vi "Main Generador N01.vi"(8 "error in":errorcluster, 11 "Network Path":string="192.168.169.1") -> (0 "error out":errorcluster, 2 "Equipo conectado":bool)   [LabVIEW 2018]
panel:
  out "current time":timestamp
  in  "Stop Button":bool
  out "Alarmas":string
  out "I3_IEE_THD%":sgl format="%.3f"
  out "I2_IEE_THD%":sgl format="%.3f"
  out "I1_IEE_THD%":sgl format="%.3f"
  out "V3_V1_IEE_THD%":sgl format="%.3f"
  out "V2_V3_IEE_THD%":sgl format="%.3f"
  out "V1_V2_IEE_THD%":sgl format="%.3f"
  out "I3_Crest_Factor":sgl format="%.3f"
  out "I2_Crest_Factor":sgl format="%.3f"
  out "I1_Crest_Factor":sgl format="%.3f"
  out "V3_V1_Crest_Factor":sgl format="%.3f"
  out "V2_V3_Crest_Factor":sgl format="%.3f"
  out "V1_V2_Crest_Factor":sgl format="%.3f"
  out "Total_Disp_PF":sgl format="%.3f"
  out "Total_True_PF":sgl format="%.3f"
  out "Total_kVA":sgl format="%.3f"
  out "Total_kVAR":sgl format="%.3f"
  out "Total_kW":sgl format="%.3f"
  out "Frequency_Hz":sgl format="%.3f"
  out "I3_Amps":sgl format="%.3f"
  out "I2_Amps":sgl format="%.3f"
  out "I1_Amps":sgl format="%.3f"
  out "V3_V1_Volts":sgl format="%.3f"
  out "V2_V3_Volts":sgl format="%.3f"
  out "V1_V2_Volts":sgl format="%.3f"
  # "G01"
  # "Generador Diesel N°1 Proa"
  # "Hora:"
  # "Fecha:"
  # "GENERAL"
  # "CALIDAD DE ENERGIA"
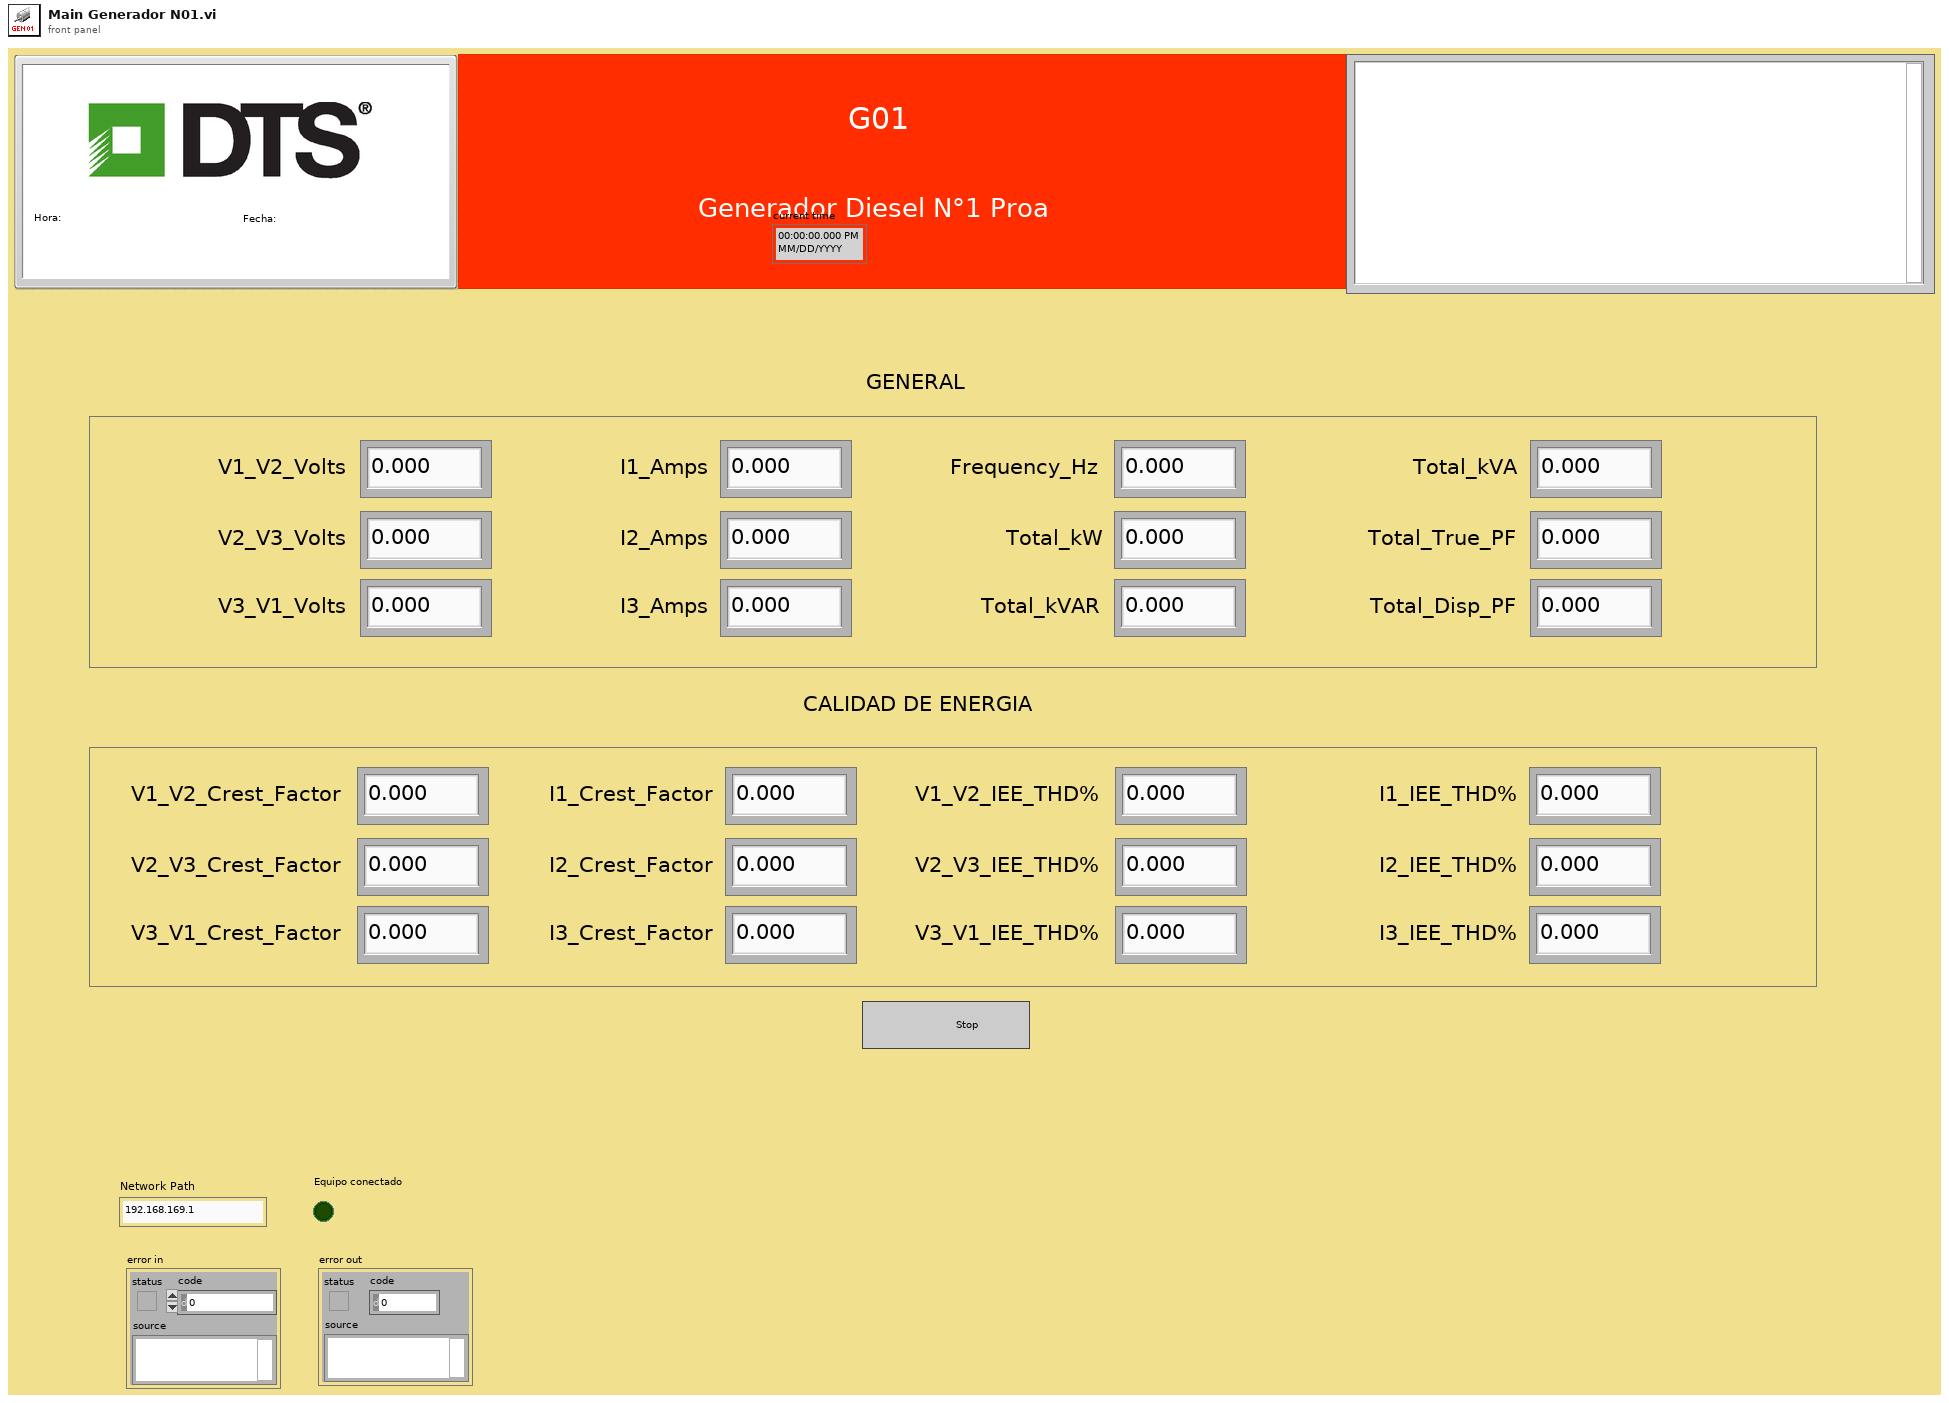
[diagram p1: front panel]
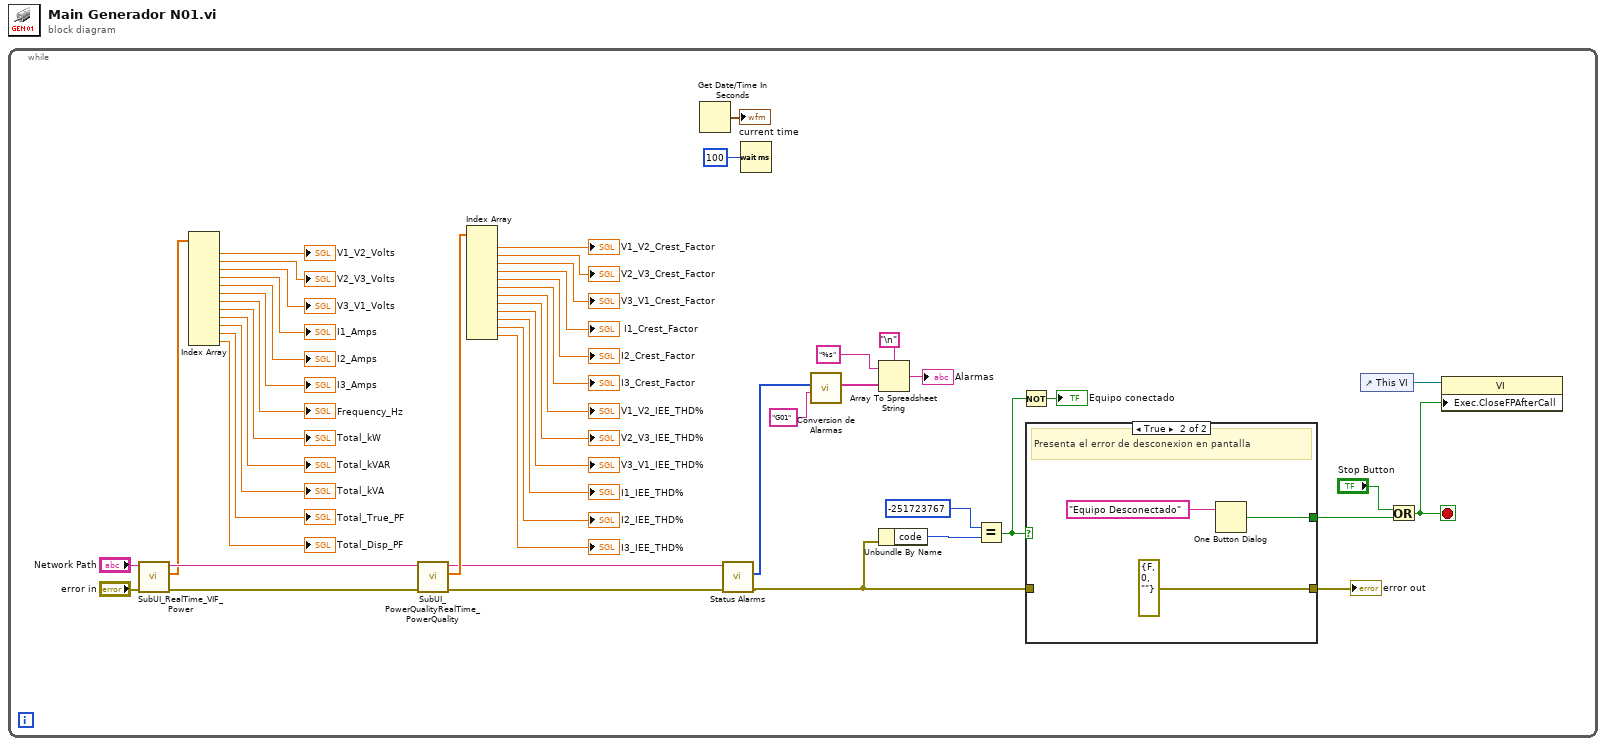
[diagram p0: block diagram]
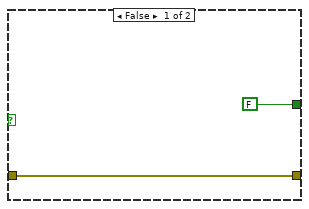
[diagram p2: hidden frame]
diagram:
  n1 = while {
    stop <- w2 stop-if-true
    n2 = call "SubUI_RealTime_VIF_Power.vi"("error in"="error in", "Network Path"="Network Path") -> ("error out"=w50:errorcluster, "Data array"=w45:sgl[], "Network Path out"=w46:string)  [unwired: 7 in]
    n3 = Index Array(array=w45) -> (element #1=→"V1_V2_Volts":sgl, element #2=→"V2_V3_Volts":sgl, element #3=→"V3_V1_Volts":sgl, element #4=→"I1_Amps":sgl, element #5=→"I2_Amps":sgl, element #6=→"I3_Amps":sgl, element #7=→"Frequency_Hz":sgl, element #8=→"Total_kW":sgl, element #9=→"Total_kVAR":sgl, element #10=→"Total_kVA":sgl, element #11=→"Total_True_PF":sgl, element #12=→"Total_Disp_PF":sgl)  [unwired: 12 in]
    n4 = call "SubUI_PowerQualityRealTime_PowerQuality.vi"("error in"=w50, "Network Path In"=w46) -> ("error out"=w13:errorcluster, "Data Array"=w32:sgl[], "Network Path Out"=w14:string)  [unwired: 7 in]
    n5 = Index Array(array=w32) -> (element #1=→"V1_V2_Crest_Factor":sgl, element #2=→"V2_V3_Crest_Factor":sgl, element #3=→"V3_V1_Crest_Factor":sgl, element #4=→"I1_Crest_Factor":sgl, element #5=→"I2_Crest_Factor":sgl, element #6=→"I3_Crest_Factor":sgl, element #7=→"V1_V2_IEE_THD%":sgl, element #8=→"V2_V3_IEE_THD%":sgl, element #9=→"V3_V1_IEE_THD%":sgl, element #10=→"I1_IEE_THD%":sgl, element #11=→"I2_IEE_THD%":sgl, element #12=→"I3_IEE_THD%":sgl)  [unwired: 12 in]
    n6 = Get Date/Time In Seconds() -> (seconds since 1Jan1904=→"current time":timestamp)
    n7 = call "Status Alarms.vi"("error in"=w13, "Network Path In"=w14) -> ("error out"=w12:errorcluster, "Data"=w10:i16[])  [unwired: 7 in, 1 out]
    n8 = Wait (ms)(milliseconds to wait=u32 100) -> ()  [unwired: 1 out]
    n9 = call "Conversion de Alarmas.vi"("Fuente"="G01", "Data Alarms"=w10) -> ("Description Alarms"=w9:string[])  [unwired: 9 in]
    n10 = Array To Spreadsheet String(delimiter (Tab)="\n", array=w9, 3:"%s" ("format string")) -> (spreadsheet string=→"Alarmas":string)
    n11 = Unbundle By Name(w12) -> ("code"=w19:i32)
    n12 = Equal?(x=-251723767, y=w19) -> (x = y?=w15:bool)
    n13 = Not(x=w15) -> (.not. x?=→"Equipo conectado":bool)
    n14 = case shown="True" w15 {
      tunnel: w12 -> [w52 _]
      tunnel: [w52 errorcluster {"status"=FALSE, "code"=0, "source"=""} ("error constant")] -> w17
      tunnel: [FALSE ("true") w53] -> w5
      frame False {
      }
      frame True {
        # "Presenta el error de desconexion en pantalla"
        n15 = One Button Dialog(message="Equipo Desconectado") -> (true=w53:bool)  [unwired: 1 in]
      }
    }
    "error out" <- w17
    n16 = control-ref of="This VI"() -> (w3:refnum<vi>)
    n17 = Or(x="Stop Button", y=w5) -> (x .or. y?=w2:bool)
    n18 = property class="VI"(reference=w3, "Exec.CloseFPAfterCall"=w2) -> ()  [unwired: 1 in, 2 out]
  }
